vi "_os_not_supported.vi"(8 "error in (no error)":errorcluster) -> (0 "error out":errorcluster, 2 "headers":string)   [LabVIEW 2020, in "advanced-http-client.lvclass"]
uses:
  advanced-http-client.lvclass
  advanced-http-client.lvclass/advanced-http-client.ctl
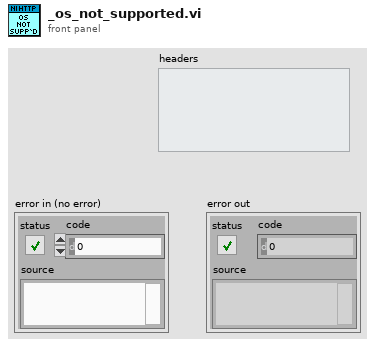
[diagram p1: front panel]
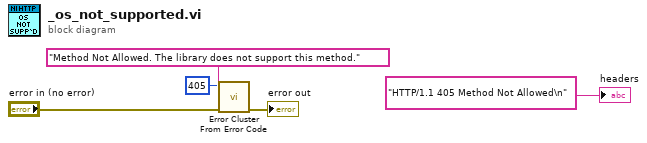
[diagram p0: block diagram]
diagram:
  n1 = call <vilib>:"Error Cluster From Error Code.vi"("error in (no error)"="error in (no error)", "error message (\"\")"="Method Not Allowed. The library does not support this method.", "error code (0)"=405) -> ("error out"=→"error out":errorcluster)  [unwired: 6 in]
  "headers" <- "HTTP/1.1 405 Method Not Allowed\n"
